vi "Create All Messages Queue.vi"(8 "error in (no error)":errorcluster) -> (0 "error out":errorcluster, 3 "Messages Queue out":T1)   [LabVIEW 2015]
uses:
  Type Definitions/All Messages Queue.ctl
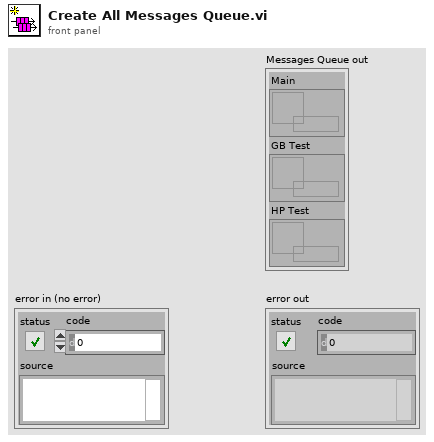
[diagram p1: front panel]
types:
  T1 = typedef "All Messages Queue.ctl" = cluster{"Main":refnum<queue>, "GB Test":refnum<queue>, "HP Test":refnum<queue>}
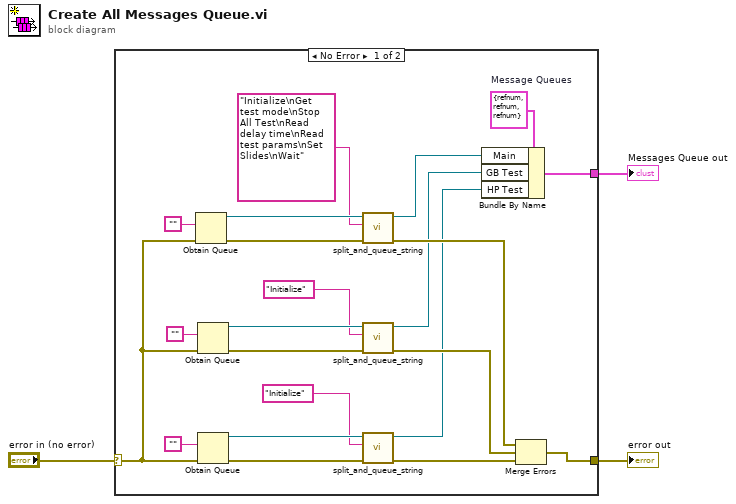
[diagram p0: block diagram]
diagram:
  n1 = case shown="No Error" "error in (no error)" {
    selector: "error in (no error)" -> [w11 w26]
    tunnel: [w22 w26] -> w3
    tunnel: [w17 _] -> w2
    frame No Error {
      w18 = T1 {"Main"=refnum, "GB Test"=refnum, "HP Test"=refnum}  # Message Queues
      n2 = Obtain Queue(element data type="", error in (no error)=w11) -> (queue out=w20:refnum<queue>, error out=w24:errorcluster)  [unwired: 3 in, 1 out]
      n3 = Obtain Queue(element data type="", error in (no error)=w11) -> (queue out=w13:refnum<queue>, error out=w12:errorcluster)  [unwired: 3 in, 1 out]
      n4 = Obtain Queue(element data type="", error in (no error)=w11) -> (queue out=w19:refnum<queue>, error out=w25:errorcluster)  [unwired: 3 in, 1 out]
      n5 = call "split_and_queue_string.vi"("error in (no error)"=w24, "program string"="Initialize\nGet test mode\nStop All Test\nRead delay time\nRead test params\nSet Slides\nWait", "queue in"=w20) -> ("error out"=w21:errorcluster, "queue out"=w8:refnum<queue>)  [unwired: 7 in]
      n6 = call "split_and_queue_string.vi"("error in (no error)"=w12, "program string"="Initialize", "queue in"=w13) -> ("error out"=w10:errorcluster, "queue out"=w7:refnum<queue>)  [unwired: 7 in]
      n7 = call "split_and_queue_string.vi"("error in (no error)"=w25, "program string"="Initialize", "queue in"=w19) -> ("error out"=w23:errorcluster, "queue out"=w9:refnum<queue>)  [unwired: 7 in]
      n8 = Bundle By Name(cluster=w18, "Main"=w8, "GB Test"=w7, "HP Test"=w9) -> (w17:T1)
      n9 = Merge Errors(w21, w10, w23) -> (w22:errorcluster)
    }
    frame Error {
    }
  }
  "error out" <- w3
  "Messages Queue out" <- w2
